vi "Get_Error_Data.vi"(0 "Error_Percentage_F_P":path, 2 "Section_E_P":string, 5 "Key_Max_Error":string, 7 "Key_Min_Error":string, 9 "Create?":bool, 11 "Error_In":errorcluster) -> (4 "Error_Data":dbl, 15 "Error_Out":errorcluster)   [LabVIEW 2023]
uses:
  <vilib>/numeric/Random Number (Range) DBL.vi
  <vilib>/Utility/config.llb/Read Key (Double).vi
  <vilib>/Utility/config.llb/NI_LVConfig.lvlib
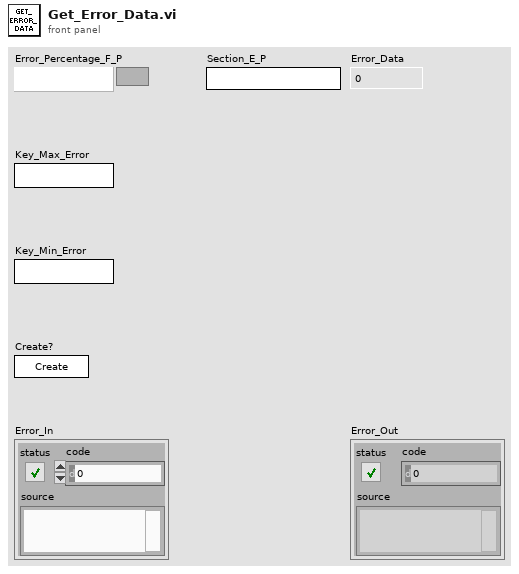
[diagram p1: front panel]
types:
  T1 = typedef "NI_LVConfig.lvlib/Config Data RefNum.ctl" = refnum<k1>
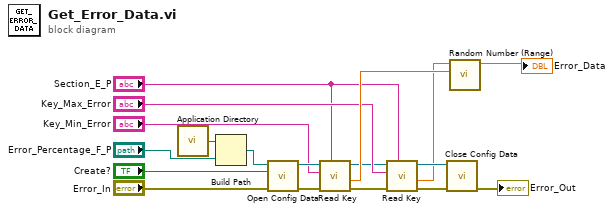
[diagram p0: block diagram]
diagram:
  n1 = call <vilib>:"Application Directory.vi"() -> ("Application Directory"=w17:path)
  n2 = Build Path(base path=w17, name or relative path="Error_Percentage_F_P") -> (appended path=w18:path)
  n3 = call <vilib>:"Open Config Data.vi"("error in (no error)"="Error_In", "create file if necessary (T)"="Create?", "configuration file path"=w18) -> ("error out"=w13:errorcluster, "refnum"=w14:T1)  [unwired: 6 in, 1 out]
  n4 = call-poly <vilib>:"Read Key.vi"("section"="Section_E_P", "error in (no error)"=w13, "key"="Key_Min_Error", "refnum"=w14) -> ("error out"=w2:errorcluster, "value"=w7:dbl, "refnum out"=w1:T1)  [unwired: 4 in, 1 out]
  n5 = call-poly <vilib>:"Read Key.vi"("section"="Section_E_P", "error in (no error)"=w2, "key"="Key_Max_Error", "refnum"=w1) -> ("error out"=w10:errorcluster, "value"=w6:dbl, "refnum out"=w9:T1)  [unwired: 4 in, 1 out]
  n6 = call <vilib>:"Close Config Data.vi"("error in (no error)"=w10, "refnum"=w9) -> ("error out"=→"Error_Out":errorcluster)  [unwired: 8 in, 1 out]
  n7 = call-poly <vilib>:"Random Number (Range).vi"("lower bound (0)"=w7, "upper bound (100)"=w6) -> ("number"=→"Error_Data":dbl)  [unwired: 9 in]
